vi "F5xxx_ZCOMP.vi"(8 "Parameter":string="R", 10 "Conn":enum16{"2-Wire", "4-Wire", "NONE"}(ring), 11 "Model":T1) -> (3 "Error Query":string)   [LabVIEW 2018]
uses:
  Models.ctl
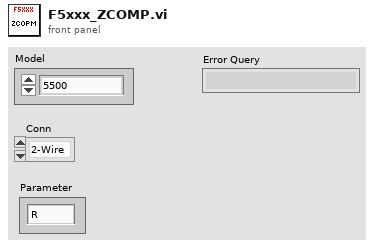
[diagram p1: front panel]
types:
  T1 = typedef "Models.ctl" = enum16{"5500", "5520", "5700", "5720", "5502", "5522", "5730"}
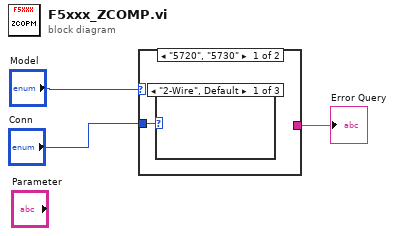
[diagram p0: block diagram]
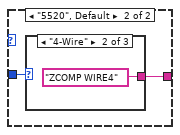
[diagram p4: hidden frame]
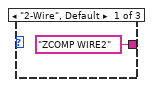
[diagram p5: hidden frame]
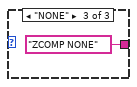
[diagram p6: hidden frame]
diagram:
  n1 = case shown="\"5720\", \"5730\"" "Model" {
    tunnel: [_ w6] -> w1
    tunnel: "Conn" -> [w4 w5]
    frame "5720", "5730" {
      n2 = case shown="\"2-Wire\", Default" w4 {
        frame "2-Wire", Default {
        }
        frame "4-Wire" {
        }
        frame "NONE" {
        }
      }
    }
    frame "5520", Default {
      n3 = case shown="\"4-Wire\"" w5 {
        tunnel: ["ZCOMP WIRE2" ("Error Query") "ZCOMP WIRE4" ("Error Query") "ZCOMP NONE" ("Error Query")] -> w6
        frame "2-Wire", Default {
        }
        frame "4-Wire" {
        }
        frame "NONE" {
        }
      }
    }
  }
  "Error Query" <- w1
